vi "Find Week of the Month.vi"(1 "Time Stamp":timestamp) -> (0 "Week of Month":i32)   [LabVIEW 2020, in "ARecurrence.lvclass"]
uses:
  ARecurrence.lvclass
  ARecurrence.lvclass/ARecurrence.ctl
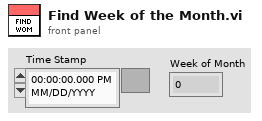
[diagram p1: front panel]
types:
  T1 = typedef "LVDateTimeRec.ctl" = cluster{"fractional second":dbl, "second":i32, "minute":i32, "hour":i32, "day of month":i32, "month":i32, "year":i32, "day of week":i32, "day of year":i32, "DST":i32}
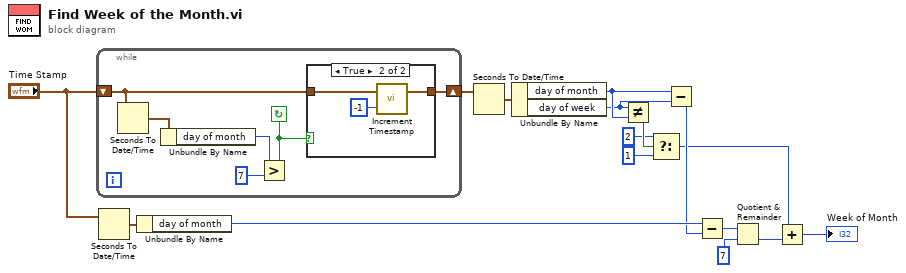
[diagram p0: block diagram]
diagram:
  n1 = while {
    shift-right: [w22] -> w16
    shift-left: "Time Stamp" -> [w21]
    stop <- w17 continue-if-true
    n2 = Seconds To Date/Time(time stamp (now)=w21) -> (date time rec=w20:T1)  [unwired: 1 in]
    n3 = Unbundle By Name(w20) -> ("day of month"=w19:i32)
    n4 = Greater?(x=w19, y=7) -> (0:w17:bool)
    n5 = case shown="True" w17 {
      tunnel: [w23 w26] -> w22
      tunnel: w21 -> [w23 w24]
      frame False {
      }
      frame True {
        n6 = call "Increment Timestamp.vi"("Days"=-1, "Time Stamp"=w24) -> ("Time Stamp out"=w26:timestamp)  [unwired: 1 in]
      }
    }
  }
  n7 = Seconds To Date/Time(time stamp (now)="Time Stamp") -> (date time rec=w13:T1)  [unwired: 1 in]
  n8 = Unbundle By Name(w13) -> ("day of month"=w7:i32)
  n9 = Seconds To Date/Time(time stamp (now)=w16) -> (date time rec=w15:T1)  [unwired: 1 in]
  n10 = Unbundle By Name(w15) -> ("day of month"=w9:i32, "day of week"=w8:i32)
  n11 = Not Equal?(x=w8, y=w9) -> (x != y?=w12:bool)
  n12 = Select(t=2, s=w12, f=1) -> (s? t:f=w2:i32)
  n13 = Subtract(x=w9, y=w8) -> (x-y=w6:i32)
  n14 = Subtract(x=w7, y=w6) -> (x-y=w5:i32)
  n15 = Quotient & Remainder(x=w5, y=7) -> (floor(x/y)=w3:i32)  [unwired: 1 out]
  n16 = Add(x=w2, y=w3) -> (x+y=→"Week of Month":i32)
